vi "NI VeriStand - Create Channel.vi"(6 "Signal ID":i32, 7 "GUID (Default Channel)":string="03D3BB99-1485-13A6-561D1F898F032919", 8 "error in":errorcluster, 9 "Faultable":bool, 10 "Channel Type":i32(ring) items=["Input", "Output"], 11 "Channel Name":string) -> (0 "error out":errorcluster, 3 "Channel Ref":refnum<k24>)   [LabVIEW 2025, in "NI_VS RuntimeConfigurationFile ScriptingAPI.lvlib"]
uses:
  NI_VS RuntimeConfigurationFile ScriptingAPI.lvlib
  NationalInstruments.VeriStand.SystemDefinitionAPI
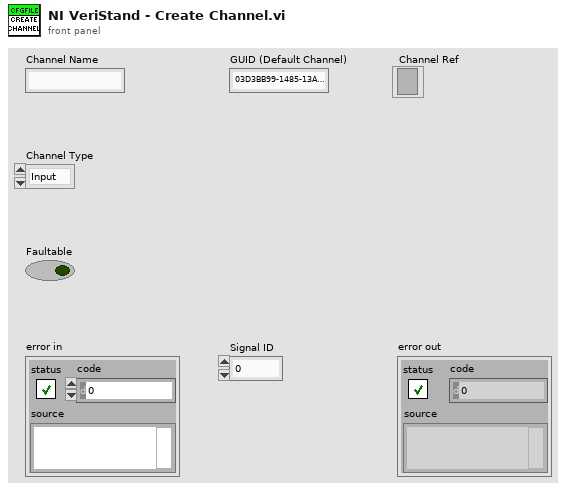
[diagram p1: front panel]
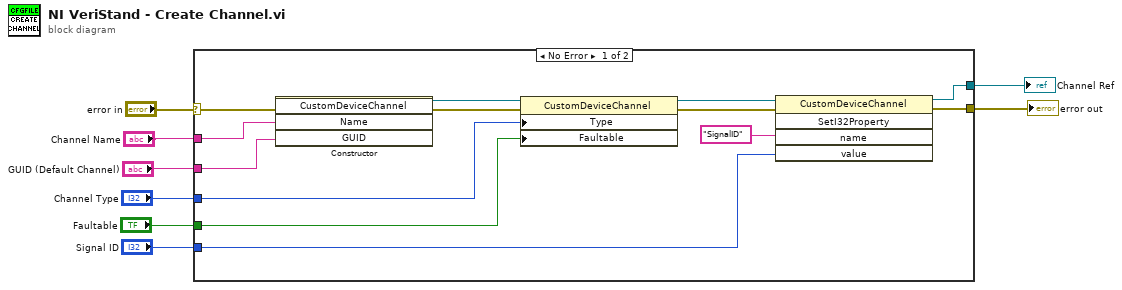
[diagram p0: block diagram]
diagram:
  n1 = case shown="No Error" "error in" {
    selector: "error in" -> [w19 w22]
    tunnel: [w20 w22] -> w8
    tunnel: "Signal ID" -> [w17 _]
    tunnel: "Channel Type" -> [w14 _]
    tunnel: "Channel Name" -> [w13 _]
    tunnel: "GUID (Default Channel)" -> [w12 _]
    tunnel: "Faultable" -> [w10 _]
    tunnel: [w9 _] -> w1
    frame No Error {
      n2 = constructor class="CustomDeviceChannel"(error in=w19, "Name"=w13, "GUID"=w12) -> (reference out=w11:refnum<k24>, error out=w18:errorcluster)  [unwired: 2 in, 3 out]
      n3 = property class="CustomDeviceChannel"(reference=w11, error in=w18, "Type"=w14, "Faultable"=w10) -> (reference out=w15:refnum<k24>, error out=w21:errorcluster)
      n4 = invoke class="CustomDeviceChannel" method="SetI32Property"(reference=w15, error in=w21, "name"="SignalID", "value"=w17) -> (reference out=w9:refnum<k24>, error out=w20:errorcluster)  [unwired: 1 in, 3 out]
    }
    frame Error {
    }
  }
  "error out" <- w8
  "Channel Ref" <- w1
